vi "1D Quadrature (VI).vi"(7 "data":variant, 8 "tolerance":dbl=1e-05, 9 "lower limit":dbl, 10 "upper limit":dbl=1.0, 11 "integrand":refnum<vi>) -> (0 "Error Out":errorcluster, 3 "result":dbl)   [LabVIEW 2021, in "Math.lvlib"]
uses:
  <vilib>/Utility/error.llb/Error Cluster From Error Code.vi
  <vilib>/ErrorRing/Error Ring.xnode
  Math.lvlib
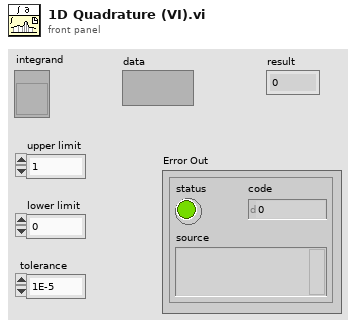
[diagram p1: front panel]
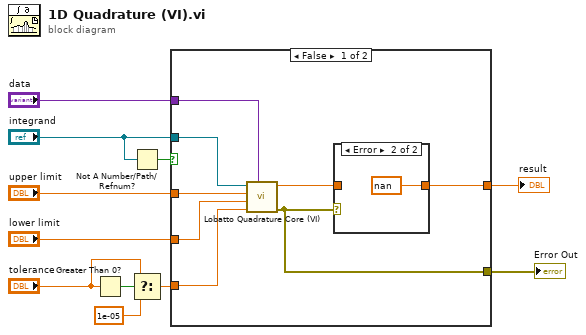
[diagram p0: block diagram]
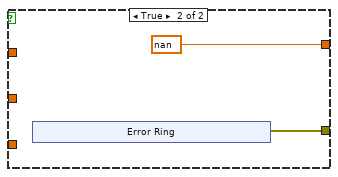
[diagram p3: hidden frame]
diagram:
  n1 = Greater Than 0?(x="tolerance") -> (x > 0?=w4:bool)
  n2 = Not A Number/Path/Refnum?(number/path/refnum="integrand") -> (NaN/Path/Refnum?=w5:bool)
  n3 = Select(t="tolerance", s=w4, f=1e-05) -> (s? t:f=w3:dbl)
  n4 = case shown="False" w5 {
    tunnel: [w19 nan] -> w8
    tunnel: "upper limit" -> [w18 _]
    tunnel: "lower limit" -> [w17 _]
    tunnel: w3 -> [w16 _]
    tunnel: "integrand" -> [w15 _]
    tunnel: "data" -> [w14 _]
    tunnel: [w12 w22] -> w1
    frame False {
      n5 = call "Lobatto Quadrature Core (VI).vi"("data"=w14, "tolerance"=w16, "lower limit"=w17, "upper limit"=w18, "f(x)"=w15) -> ("error out"=w12:errorcluster, "result"=w13:dbl)  [unwired: 5 in]
      n6 = case shown="Error" w12 {
        tunnel: w13 -> [w20 _]
        tunnel: [w20 nan] -> w19
        frame No Error {
        }
        frame Error {
        }
      }
    }
    frame True {
      n7 = xnode "Error Ring"() -> ("error out"=w22:errorcluster)
    }
  }
  "result" <- w8
  "Error Out" <- w1
